vi "Get ControlPacket Bytes.vi"(6 "Validate? (F)":bool, 8 "error in (no error)":errorcluster, 11 "ControlPacket":refnum<class "ControlPacket.lvclass">) -> (0 "error out":errorcluster, 1 "Packet invalid":bool, 2 "Bytes Stream":u8[](array[numeric]) format="%08b", 3 "ControlPacket dup":refnum<class "ControlPacket.lvclass">)   [LabVIEW 2013, in "MQTT_Control_Packets.lvlib" / "ControlPacket.lvclass"]
uses:
  ControlPacket.lvclass
  ControlPacket.lvclass/ControlPacket.ctl
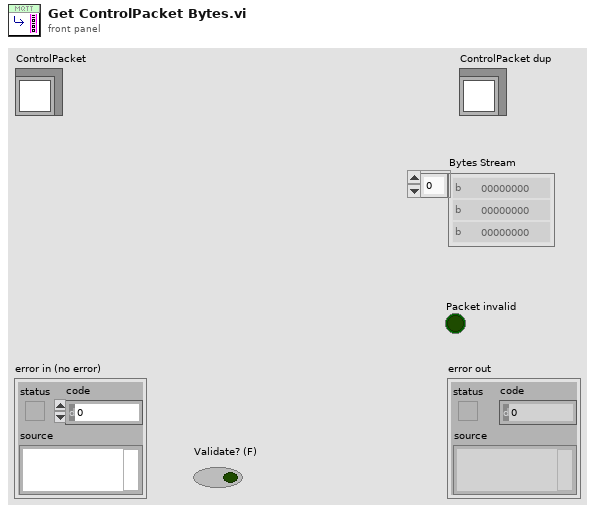
[diagram p1: front panel]
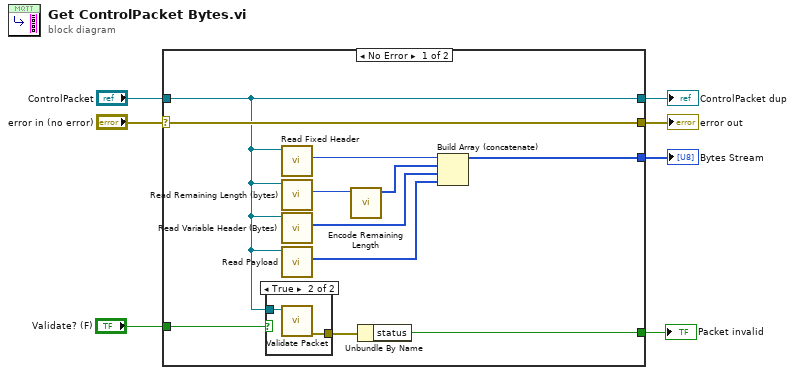
[diagram p0: block diagram]
diagram:
  n1 = case shown="No Error" "error in (no error)" {
    selector: "error in (no error)" -> [w18 w22]
    tunnel: [w18 w22] -> w6
    tunnel: [w11 w21] -> w4
    tunnel: "ControlPacket" -> [w11 w21]
    tunnel: "Validate? (F)" -> [w10 _]
    tunnel: [w12 _] -> w2
    tunnel: [w8 _] -> w1
    frame No Error {
      n2 = case shown="True" w10 {
        tunnel: w11 -> [_ w20]
        tunnel: [_ w19] -> w9
        frame False {
        }
        frame True {
          n3 = call "Validate Packet.vi"("ControlPacket in"=w20) -> ("error out"=w19:errorcluster)  [unwired: 9 in, 1 out]
        }
      }
      n4 = call "Read Fixed Header.vi"("ControlPacket in"=w11) -> ("Fixed Header"=w17:u8)  [unwired: 9 in, 1 out]
      n5 = call "Read Remaining Length (bytes).vi"("ControlPacket in"=w11) -> ("Remaining Length (bytes)"=w16:u32)  [unwired: 8 in, 2 out]
      n6 = call "Read Variable Header (Bytes).vi"("ControlPacket in"=w11) -> ("Variable Header (Bytes)"=w14:u8[])  [unwired: 9 in, 1 out]
      n7 = call "Read Payload.vi"("ControlPacket in"=w11) -> ("Payload"=w13:u8[])  [unwired: 9 in, 1 out]
      n8 = call "Encode Remaining Length.vi"("Remaining Length (bytes)"=w16) -> ("Encoded Remaining Length"=w15:u8[])  [unwired: 9 in, 1 out]
      n9 = Unbundle By Name(w9) -> ("status"=w8:bool)
      n10 = Build Array (concatenate)(w17, w15, w14, w13) -> (w12:u8[])
    }
    frame Error {
    }
  }
  "error out" <- w6
  "ControlPacket dup" <- w4
  "Bytes Stream" <- w2
  "Packet invalid" <- w1
